vi "lv-ros-bridge_READ.vi"(8 "error in (no error)":errorcluster, 9 "Topic to subscribe":string="/", 10 "rosbridge port":u16=9090, 11 "rosbridge server IP":string="192.168.164.128") -> (0 "error out":errorcluster)   [LabVIEW 2015]
uses:
  <vilib>/MediaMongrels Ltd/WebSockets/WebSockets/WebSockets.lvlib
panel:
  out "value 4":T1
  in  "szablon CMD_VEL":T1
  out "Data 2":string
  out "Opcode 2":u8
  in  "szablon 2":T2
  in  "stop 2":bool
  out "value 3":T2
  in  "rosbridge server IP 2":string="192.168.164.128"
  in  "rosbridge port 2":u16=9090
  in  "error in (no error) 2":errorcluster
  out "error out 2":errorcluster
  in  "Topic to subscribe 2":string="/"
  out "value 2":T3
  in  "STEERING":T3
  out "value":T2
  in  "szablon":T2
  out "Opcode":u8
  out "Data":string
  in  "stop":bool
  # "e"
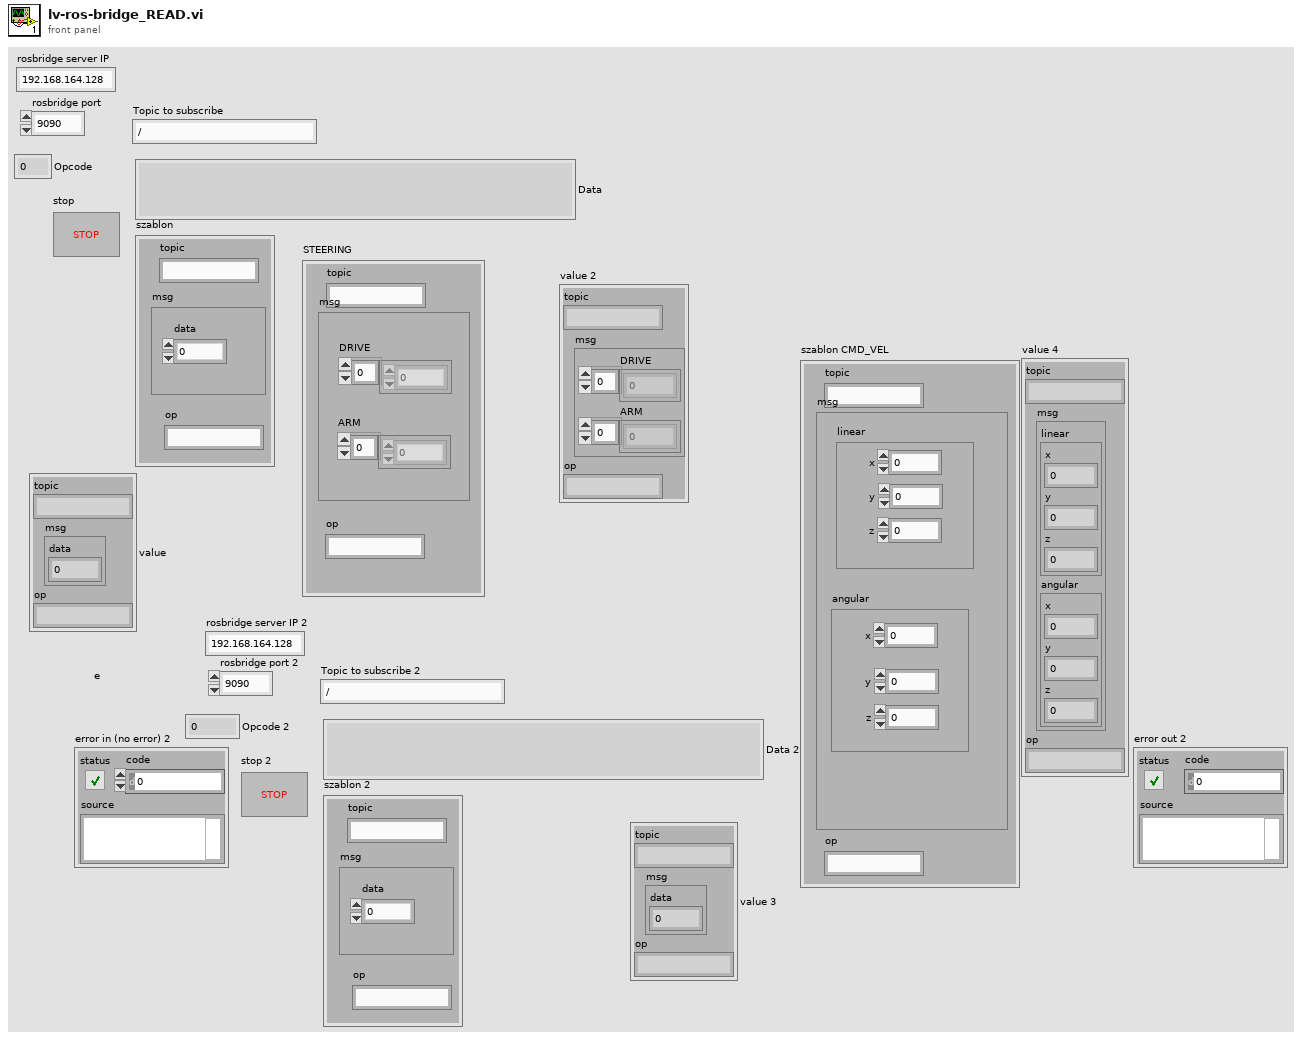
[diagram p1: front panel]
types:
  T1 = cluster{"topic":string, "msg":cluster{"linear":cluster{"x":dbl, "y":dbl, "z":dbl}, "angular":cluster{"x":dbl, "y":dbl, "z":dbl}}, "op":string}
  T2 = cluster{"topic":string, "msg":cluster{"data":i16}, "op":string}
  T3 = cluster{"topic":string, "msg":cluster{"DRIVE":i16[], "ARM":i8[]}, "op":string}
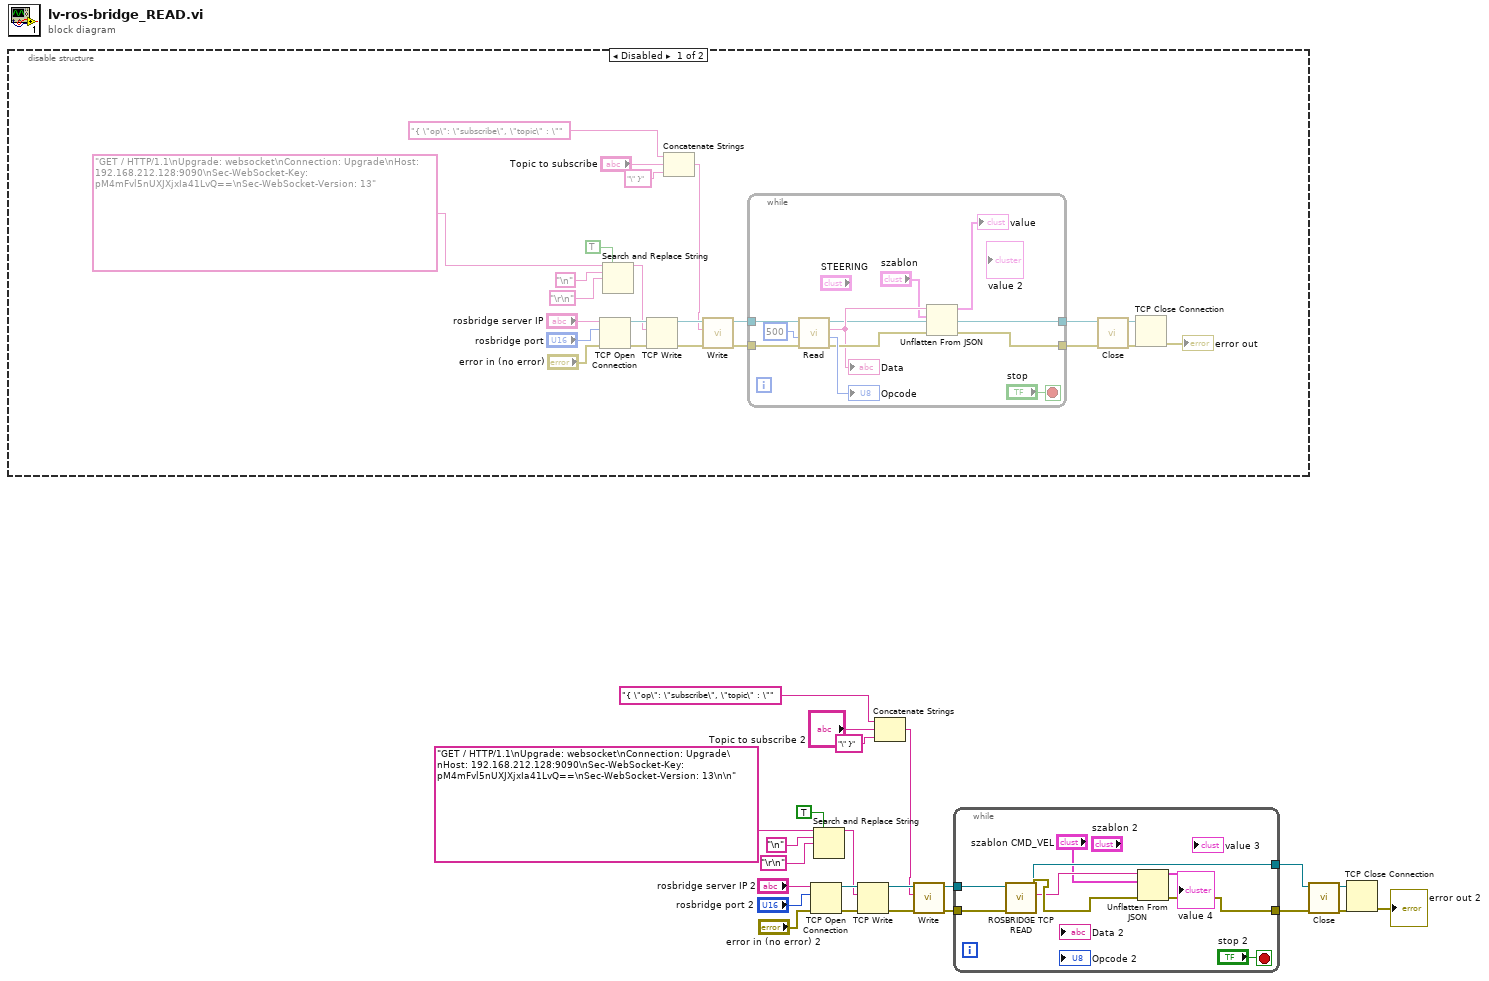
[diagram p0: block diagram]
diagram:
  n1 = disable-structure shown="Disabled" {
    frame Disabled {
      n2 = TCP Open Connection(address="rosbridge server IP", remote port or service name="rosbridge port", error in (no error)="error in (no error)") -> (connection ID=w44:refnum<k5>, error out=w43:errorcluster)  [unwired: 2 in]
      n3 = Search and Replace String(replace all?=TRUE ("replace all? (F)"), input string="GET / HTTP/1.1\nUpgrade: websocket\nConnection: Upgrade\nHost: 192.168.212.128:9090\nSec-WebSocket-Key: pM4mFvl5nUXJXjxIa41LvQ==\nSec-WebSocket-Version: 13", search string="\n", replace string="\r\n") -> (result string=w29:string)  [unwired: 4 in, 3 out]
      n4 = TCP Write(connection ID=w44, data in=w29, error in (no error)=w43) -> (connection ID out=w40:refnum<k5>, error out=w39:errorcluster)  [unwired: 1 in, 1 out]
      n5 = Concatenate Strings("{ \"op\": \"subscribe\", \"topic\" : \"", "Topic to subscribe", "\" }") -> (w27:string)
      n6 = call <vilib>:"Write.vi"("error in (no error)"=w39, "Data"=w27, "WebSocket Connection in"=w40) -> ("error out"=w35:errorcluster, "WebSocket Connection out"=w36:refnum<k5>)  [unwired: 7 in]
      n7 = while {
        tunnel: [w50] -> w38
        tunnel: [w49] -> w37
        tunnel: w36 -> [w57]
        tunnel: w35 -> [w56]
        stop <- "stop" stop-if-true
        n8 = call <vilib>:"Read.vi"("error in (no error)"=w56, "timeout ms (5000)"=500, "WebSocket Connection in"=w57) -> ("error out"=w53:errorcluster, "Opcode"=→"Opcode":u8, "Data"=w52:string, "WebSocket Connection out"=w50:refnum<k5>)  [unwired: 5 in]
        "Data" <- w52
        n9 = Unflatten From JSON(JSON string=w52, type and defaults="szablon", error in (no error)=w53) -> (value=→"value":T2, error out=w49:errorcluster)  [unwired: 4 in]
      }
      n10 = call <vilib>:"Close.vi"("error in (no error)"=w37, "WebSocket Connection in"=w38) -> ("error out"=w41:errorcluster, "WebSocket Connection in"=w42:refnum<k5>)  [unwired: 8 in]
      n11 = TCP Close Connection(connection ID=w42, error in (no error)=w41) -> (error out=→"error out":errorcluster)  [unwired: 1 in, 1 out]
    }
    frame Enabled {
    }
  }
  n12 = TCP Open Connection(address="rosbridge server IP 2", remote port or service name="rosbridge port 2", error in (no error)="error in (no error) 2") -> (connection ID=w21:refnum<k5>, error out=w20:errorcluster)  [unwired: 2 in]
  n13 = Search and Replace String(replace all?=TRUE ("replace all? (F)"), input string="GET / HTTP/1.1\nUpgrade: websocket\nConnection: Upgrade\nHost: 192.168.212.128:9090\nSec-WebSocket-Key: pM4mFvl5nUXJXjxIa41LvQ==\nSec-WebSocket-Version: 13\n\n", search string="\n", replace string="\r\n") -> (result string=w6:string)  [unwired: 4 in, 3 out]
  n14 = TCP Write(connection ID=w21, data in=w6, error in (no error)=w20) -> (connection ID out=w17:refnum<k5>, error out=w16:errorcluster)  [unwired: 1 in, 1 out]
  n15 = Concatenate Strings("{ \"op\": \"subscribe\", \"topic\" : \"", "Topic to subscribe 2", "\" }") -> (w4:string)
  n16 = call <vilib>:"Write.vi"("error in (no error)"=w16, "Data"=w4, "WebSocket Connection in"=w17) -> ("error out"=w13:errorcluster, "WebSocket Connection out"=w14:refnum<k5>)  [unwired: 7 in]
  n17 = while {
    tunnel: [w65] -> w15
    tunnel: w14 -> [w64]
    tunnel: w13 -> [w63]
    tunnel: [w60] -> w1
    stop <- "stop 2" stop-if-true
    n18 = call "ROSBRIDGE TCP READ.vi"("error in (no error)"=w63, "TCP Network Connection in"=w64) -> ("error out"=w62:errorcluster, "String out"=w61:string, "TCP Network Connection out"=w60:refnum<k5>)  [unwired: 7 in]
    n19 = Unflatten From JSON(JSON string=w61, type and defaults="szablon CMD_VEL", error in (no error)=w62) -> (value=→"value 4":T1, error out=w65:errorcluster)  [unwired: 4 in]
  }
  n20 = call <vilib>:"Close.vi"("error in (no error)"=w15, "WebSocket Connection in"=w1) -> ("error out"=w18:errorcluster, "WebSocket Connection in"=w19:refnum<k5>)  [unwired: 8 in]
  n21 = TCP Close Connection(connection ID=w19, error in (no error)=w18) -> (error out=→"error out 2":errorcluster)  [unwired: 1 in, 1 out]
